vi "Camera_Convert Camera Settings General to Detailed.vi"(9 "Camera Settings":T2 {"Saturation" min=0 max=100 step=1; "Sharpness" min=0 max=100 step=1; "Brightness" min=0 max=100 step=1; "Exposure (%)" min=0.0 max=100.0 step=1.0}, 11 "Detailed Values":T1) -> (3 "Detailed Values Out":T1)   [LabVIEW 2017, in "VisionSystem.lvlib"]
uses:
  VisionSystem.lvlib
  <vilib>/Rock Robotics/WPI/Camera/WPI_CameraImageSize.ctl
  <vilib>/Rock Robotics/WPI/Camera/WPI_CameraFrameRate.ctl
  <vilib>/Rock Robotics/WPI/Camera/WPI_CameraWhite Balance Values.ctl
  <vilib>/Rock Robotics/WPI/Camera/WPI_CameraExposure Values.ctl
  TypeDefs/Cluster_Camera Settings.ctl
  <vilib>/Rock Robotics/WPI/Camera/WPI_CameraSettings Control.ctl
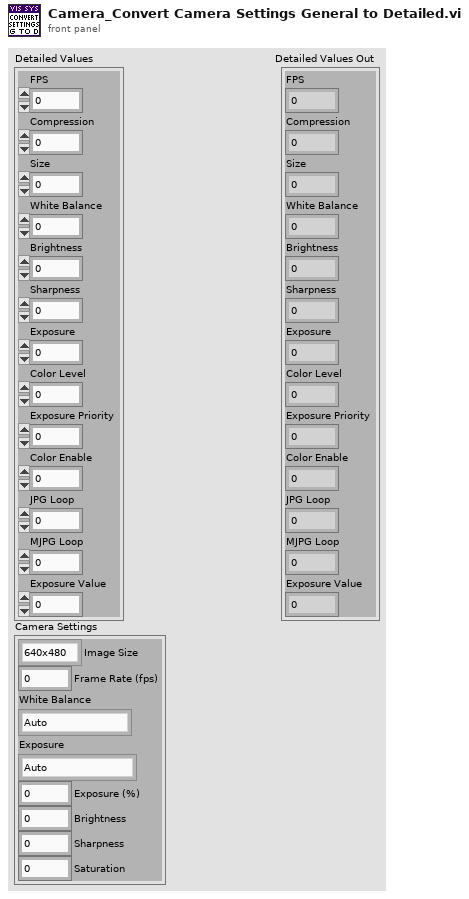
[diagram p1: front panel]
types:
  T1 = typedef "WPI_CameraSettings Control.ctl" = cluster{"FPS":i32, "Compression":i32, "Size":i32, "White Balance":i32, "Brightness":i32, "Sharpness":i32, "Exposure":i32, "Color Level":i32, "Exposure Priority":i32, "Color Enable":i32, "JPG Loop":i32, "MJPG Loop":i32, "Exposure Value":i32}
  T2 = typedef "Cluster_Camera Settings.ctl" = cluster{"Image Size":T3, "Frame Rate (fps)":T4, "White Balance":T5, "Exposure":T6, "Exposure (%)":dbl, "Brightness":i32, "Sharpness":i32, "Saturation":i32}
  T3 = typedef "WPI_CameraImageSize.ctl" = enum16{"640x480", "320x240", "160x120", "Custom"}
  T4 = typedef "WPI_CameraFrameRate.ctl" = u32
  T5 = typedef "WPI_CameraWhite Balance Values.ctl" = enum16{"Auto", "Fixed indoor", "Fixed outdoor 1", "Fixed outdoor 2", "Fixed fluorescent 1", "Fixed fluorescent 2", "Hold current", "Custom"}
  T6 = typedef "WPI_CameraExposure Values.ctl" = enum16{"Auto", "Flicker-free 50 Hz", "Flicker-free 60 Hz", "Hold current", "Custom"}
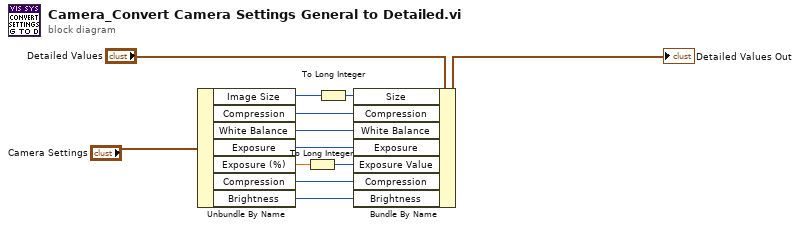
[diagram p0: block diagram]
diagram:
  n1 = Unbundle By Name("Camera Settings") -> ("Image Size"=w9:T3, "Compression"=w7:i32, "White Balance"=w6:T5, "Exposure"=w5:T6, "Exposure (%)"=w2:dbl, "Compression"=w3:i32, "Brightness"=w4:i32)
  n2 = To Long Integer(number=w2) -> (32bit integer=w1:i32)
  n3 = To Long Integer(number=w9) -> (32bit integer=w8:i32)
  n4 = Bundle By Name(cluster="Detailed Values", "Size"=w8, "Compression"=w7, "White Balance"=w6, "Exposure"=w5, "Exposure Value"=w1, "Compression"=w3, "Brightness"=w4) -> (→"Detailed Values Out":T1)
